vi "Shoot test.vi"(0 "Shoot":bool, 1 "Current Angle":dbl=154.45246409191577, 2 "Current Motor SetPoint":dbl=-0.055756046742338715) -> (5 "New Motor Setpoint":dbl=-0.055756046742338715)   [LabVIEW 2013]
uses:
  Robot Global Data.vi
panel:
  in  "Coast Bias":dbl=0.3 format="%#_13g"
  in  "Motor Bias":dbl=1.0
  out "Cycle time":u32=605
  out "Shoot time":u32=284
  out "Meas. Angle":dbl(graph)=159.45935903131544
  out "Encoder Rate (deg/sec)":dbl=399.75071225071224
  out "Meas. Speed":cluster{i32, dbl}(graph)
  out "Error":dbl=0.5
  in  "Speed Gain":dbl=0.003 step=0.0005
  in  "Measured Rate":dbl
  in  "Desired Rate":dbl=50.0
  in  "Launch Angle":dbl=161.0
  # "This should be 1\nwhen tested !!!"
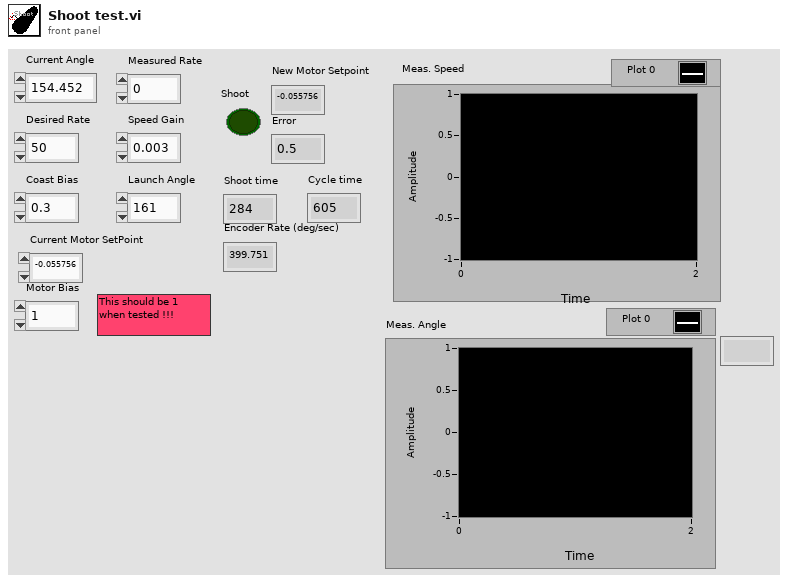
[diagram p1: front panel]
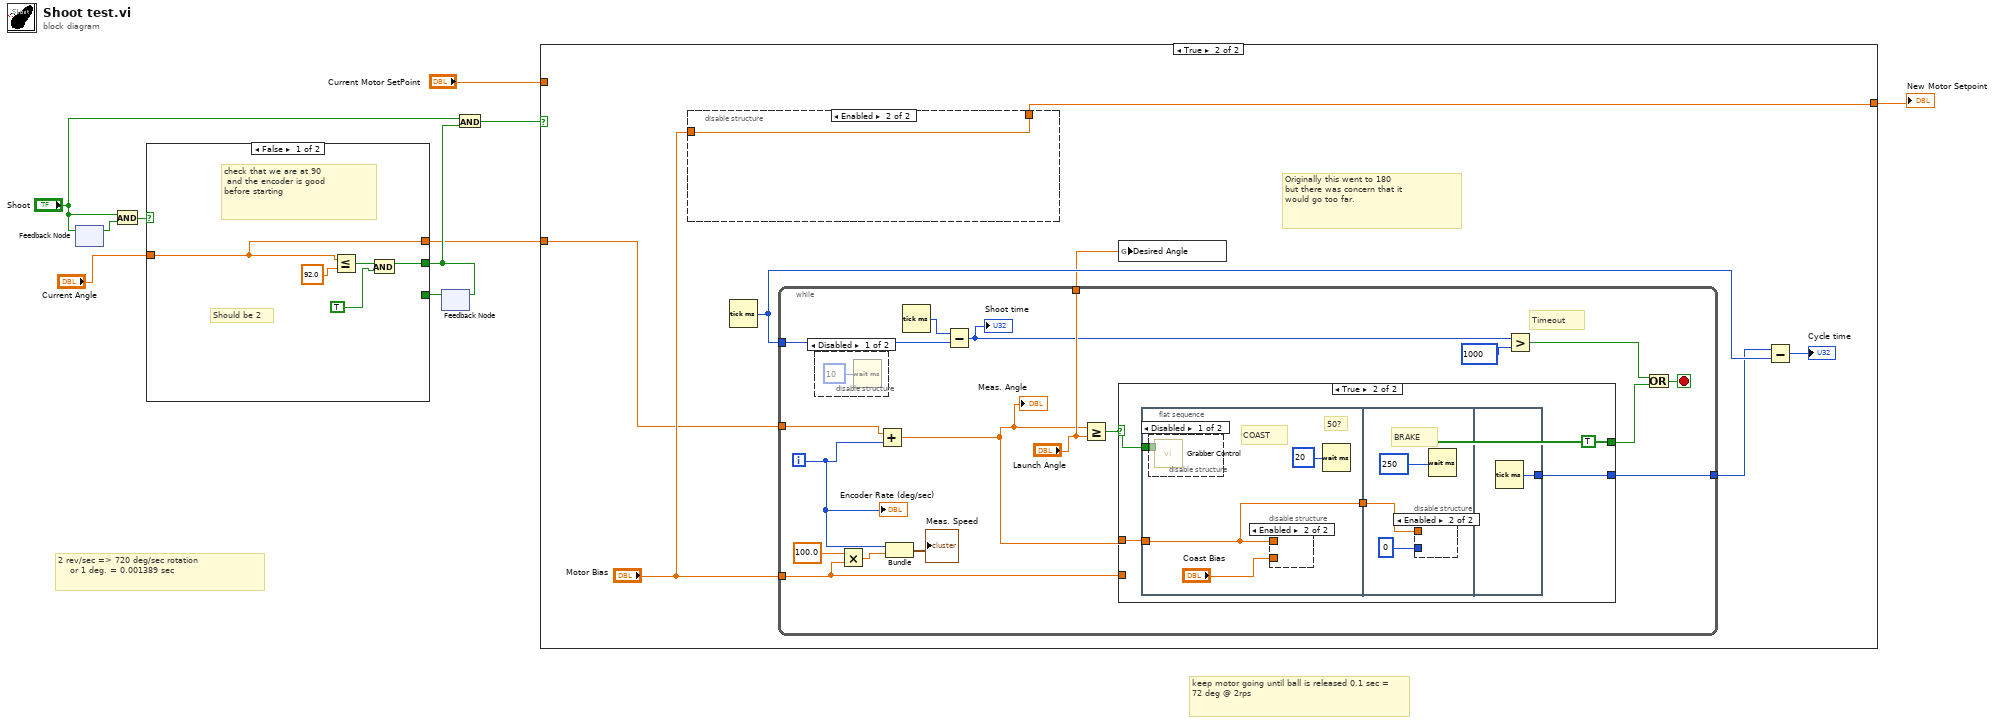
[diagram p0: block diagram]
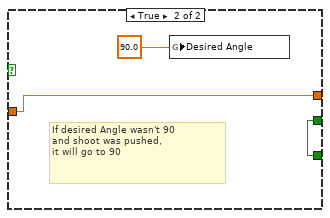
[diagram p2: hidden frame]
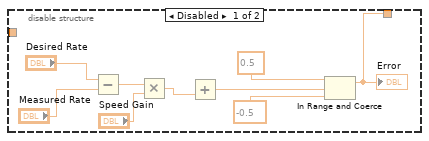
[diagram p4: hidden frame]
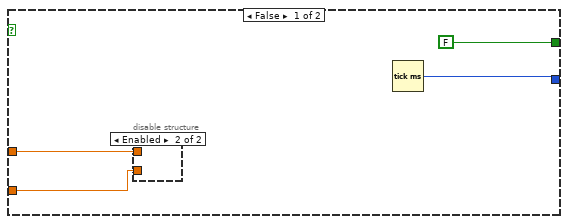
[diagram p6: hidden frame]
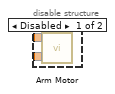
[diagram p7: hidden frame]
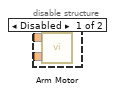
[diagram p8: hidden frame]
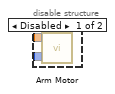
[diagram p10: hidden frame]
diagram:
  # "keep motor going until ball is released 0.1 sec = 72 deg @ 2rps"
  # "2 rev/sec => 720 deg/sec rotation\n    or 1 deg. = 0.001389 sec"
  n1 = feedback-in #1("Shoot") -> ()
  n2 = feedback #1() -> (w8:bool)  [unwired: 1 in]
  n3 = And(x="Shoot", y=w8) -> (x .and. y?=w7:bool)
  n4 = feedback #2() -> (w3:bool)  [unwired: 1 in]
  n5 = case shown="False" w7 {
    tunnel: [w13 w18] -> w4
    tunnel: w3 -> [_ w18]
    tunnel: [w12 w16] -> w2
    tunnel: "Current Angle" -> [w12 w16]
    frame False {
      # "Should be 2"
      # "check that we are at 90\n and the encoder is good\nbefore starting"
      n6 = Less Or Equal?(x=w12, y=92.0) -> (x <= y?=w14:bool)
      n7 = And(x=w14, y=TRUE) -> (x .and. y?=w13:bool)
    }
    frame True {
      # "If desired Angle wasn't 90\nand shoot was pushed,  \nit will go to 90"
      n8 = global write "Robot Global Data.vi" "Desired Angle"(90.0 ("Desired Angle")) -> ()
    }
  }
  n9 = feedback-in #2(w4) -> ()
  n10 = And(x="Shoot", y=w4) -> (x .and. y?=w6:bool)
  n11 = case shown="True" w6 {
    tunnel: "Current Motor SetPoint" -> [w19 _]
    tunnel: [w19 w23] -> w9
    tunnel: w2 -> [_ w20]
    frame False {
    }
    frame True {
      # "Originally this went to 180\nbut there was concern that it \nwould go too far."
      n12 = disable-structure shown="Enabled" {
        disable-tunnel: [w30 w36] -> w23
        disable-tunnel: "Motor Bias" -> [_ w36]
        frame Disabled {
          n13 = Subtract(x="Desired Rate", y="Measured Rate") -> (x-y=w35:dbl)
          n14 = Multiply(x=w35, y="Speed Gain") -> (x*y=w28:dbl)
          n15 = Add(y=w28) -> (x+y=w29:dbl)  [unwired: 1 in]
          n16 = In Range and Coerce(upper limit=0.5, x=w29, lower limit=-0.5) -> (coerced(x)=w30:dbl)  [unwired: 1 out]
          "Error" <- w30
        }
        frame Enabled {
        }
      }
      n17 = Tick Count (ms)() -> (millisecond timer value=w26:u32)
      n18 = while {
        tunnel: w26 -> [w51]
        tunnel: [w38] -> w24
        tunnel: "Motor Bias" -> [w37]
        tunnel: ["Launch Angle"] -> w21
        tunnel: w20 -> [w45]
        i -> [w41]
        stop <- w49 stop-if-true
        # "Timeout"
        n19 = disable-structure shown="Disabled" {
          frame Disabled {
            n20 = Wait (ms)(milliseconds to wait=u32 10) -> ()  [unwired: 1 out]
          }
          frame Enabled {
          }
        }
        n21 = Multiply(x=100.0, y=w37) -> (x*y=w43:dbl)
        n22 = Add(x=w45, y=w41) -> (x+y=w46:dbl)
        "Meas. Angle" <- w46
        n23 = Bundle(w41, w43) -> (→"Meas. Speed":cluster{i32, dbl})  [unwired: 1 in]
        n24 = Tick Count (ms)() -> (millisecond timer value=w52:u32)
        n25 = Subtract(x=w52, y=w51) -> (x-y=w40:u32)
        "Shoot time" <- w40
        n26 = Greater Or Equal?(x=w46, y="Launch Angle") -> (x >= y?=w48:bool)
        n27 = case shown="True" w48 {
          selector: w48 -> [_ w65]
          tunnel: w46 -> [w57 w64]
          tunnel: w37 -> [w58 _]
          tunnel: [FALSE TRUE] -> w39
          tunnel: [w55 w61] -> w38
          frame False {
            n28 = disable-structure shown="Enabled" {
              disable-tunnel: w57 -> [w60 _]
              disable-tunnel: w58 -> [w59 _]
              frame Disabled {
                n29 = call "Arm Motor.vi"("Motor input"=w59, "Current angle (deg)"=w60) -> ()  [unwired: 1 in]
              }
              frame Enabled {
              }
            }
            n30 = Tick Count (ms)() -> (millisecond timer value=w55:u32)
          }
          frame True {
            n31 = flat-sequence {
              tunnel: w65 -> [w69]
              tunnel: w64 -> [w66]
              tunnel: [w66] -> w63
              tunnel: w63 -> [w74]
              tunnel: [w78] -> w61
              frame #0 {
                # "COAST"
                # "50?"
                n32 = disable-structure shown="Disabled" {
                  disable-tunnel: w69 -> [w72 _]
                  frame Disabled {
                    n33 = call "Grabber Control.vi"("Open Claws"=w72) -> ()  [unwired: 2 in]
                  }
                  frame Enabled {
                  }
                }
                n34 = disable-structure shown="Enabled" {
                  disable-tunnel: w66 -> [w71 _]
                  disable-tunnel: "Coast Bias" -> [w70 _]
                  frame Disabled {
                    n35 = call "Arm Motor.vi"("Motor input"=w70, "Current angle (deg)"=w71) -> ()  [unwired: 1 in]
                  }
                  frame Enabled {
                  }
                }
                n36 = Wait (ms)(milliseconds to wait=u32 20) -> ()  [unwired: 1 out]
              }
              frame #1 {
                # "BRAKE"
                n37 = disable-structure shown="Enabled" {
                  disable-tunnel: w74 -> [w77 _]
                  disable-tunnel: 0 -> [w76 _]
                  frame Disabled {
                    n38 = call "Arm Motor.vi"("Motor input"=w76, "Current angle (deg)"=w77) -> ()  [unwired: 1 in]
                  }
                  frame Enabled {
                  }
                }
                n39 = Wait (ms)(milliseconds to wait=u32 250) -> ()  [unwired: 1 out]
              }
              frame #2 {
                n40 = Tick Count (ms)() -> (millisecond timer value=w78:u32)
              }
            }
          }
        }
        n41 = Greater?(x=w40, y=u32 1000) -> (0:w50:bool)
        n42 = Or(x=w50, y=w39) -> (x .or. y?=w49:bool)
        "Encoder Rate (deg/sec)" <- w41
      }
      n43 = global write "Robot Global Data.vi" "Desired Angle"(w21) -> ()
      n44 = Subtract(x=w24, y=w26) -> (x-y=→"Cycle time":u32)
    }
  }
  "New Motor Setpoint" <- w9
